vi "viserverUserAccess_getUserNamesSymbols.vi"(0 "ACL in":refnum<k20>, 5 "principal array in":T1[](array[typedef]) {"principal"."ID"."b7" format="%02x"; "principal"."ID"."b6" format="%02x"; "principal"."ID"."b5" format="%02x"; "principal"."ID"."b4" format="%02x"; "principal"."ID"."b3" format="%02x"; "principal"."ID"."b2" format="%02x"; "principal"."ID"."b1" format="%02x"; "principal"."ID"."b0" format="%02x"; "principal"."ID"."b15" format="%02x"; "principal"."ID"."b14" format="%02x"; "principal"."ID"."b13" format="%02x"; "principal"."ID"."b12" format="%02x"; "principal"."ID"."b11" format="%02x"; "principal"."ID"."b10" format="%02x"; "principal"."ID"."b9" format="%02x"; "principal"."ID"."b8" format="%02x"; "domain"."ID"."b7" format="%02x"; "domain"."ID"."b6" format="%02x"; "domain"."ID"."b5" format="%02x"; "domain"."ID"."b4" format="%02x"; "domain"."ID"."b3" format="%02x"; "domain"."ID"."b2" format="%02x"; "domain"."ID"."b1" format="%02x"; "domain"."ID"."b0" format="%02x"; "domain"."ID"."b15" format="%02x"; "domain"."ID"."b14" format="%02x"; "domain"."ID"."b13" format="%02x"; "domain"."ID"."b12" format="%02x"; "domain"."ID"."b11" format="%02x"; "domain"."ID"."b10" format="%02x"; "domain"."ID"."b9" format="%02x"; "domain"."ID"."b8" format="%02x"}, 11 "error in (no error)":errorcluster) -> (4 "ACL out":refnum<k20>, 6 "principal array out":T1[](array[typedef]) {"principal"."ID"."b7" format="%02x"; "principal"."ID"."b6" format="%02x"; "principal"."ID"."b5" format="%02x"; "principal"."ID"."b4" format="%02x"; "principal"."ID"."b3" format="%02x"; "principal"."ID"."b2" format="%02x"; "principal"."ID"."b1" format="%02x"; "principal"."ID"."b0" format="%02x"; "principal"."ID"."b15" format="%02x"; "principal"."ID"."b14" format="%02x"; "principal"."ID"."b13" format="%02x"; "principal"."ID"."b12" format="%02x"; "principal"."ID"."b11" format="%02x"; "principal"."ID"."b10" format="%02x"; "principal"."ID"."b9" format="%02x"; "principal"."ID"."b8" format="%02x"; "domain"."ID"."b7" format="%02x"; "domain"."ID"."b6" format="%02x"; "domain"."ID"."b5" format="%02x"; "domain"."ID"."b4" format="%02x"; "domain"."ID"."b3" format="%02x"; "domain"."ID"."b2" format="%02x"; "domain"."ID"."b1" format="%02x"; "domain"."ID"."b0" format="%02x"; "domain"."ID"."b15" format="%02x"; "domain"."ID"."b14" format="%02x"; "domain"."ID"."b13" format="%02x"; "domain"."ID"."b12" format="%02x"; "domain"."ID"."b11" format="%02x"; "domain"."ID"."b10" format="%02x"; "domain"."ID"."b9" format="%02x"; "domain"."ID"."b8" format="%02x"}, 8 "User/group names":string[](array[string]), 10 "User/group access symbols":i32[](array[numeric]), 15 "error out":errorcluster)   [LabVIEW 2020]
uses:
  <vilib>/Platform/security/user/NI_Security Qualified Domain-Principal Pair.ctl
  <vilib>/Platform/security/user/NI_Security Domain.ctl
  <vilib>/Platform/security/user/NI_Security Identifier.ctl
  <vilib>/Platform/security/user/NI_Security Principal.ctl
  <vilib>/Platform/security/user/NI_Security PrincipalType.ctl
  <vilib>/Platform/SharedPrefPage_SubVIs/viServerUserAccess_user_group_enum.ctl
  <vilib>/Platform/security/user/NI_Security AccessRights_CloseRef.vi
  <vilib>/Platform/security/user/NI_Security ACE_CloseRef.vi
  <resource>/objmgr/Security.rc
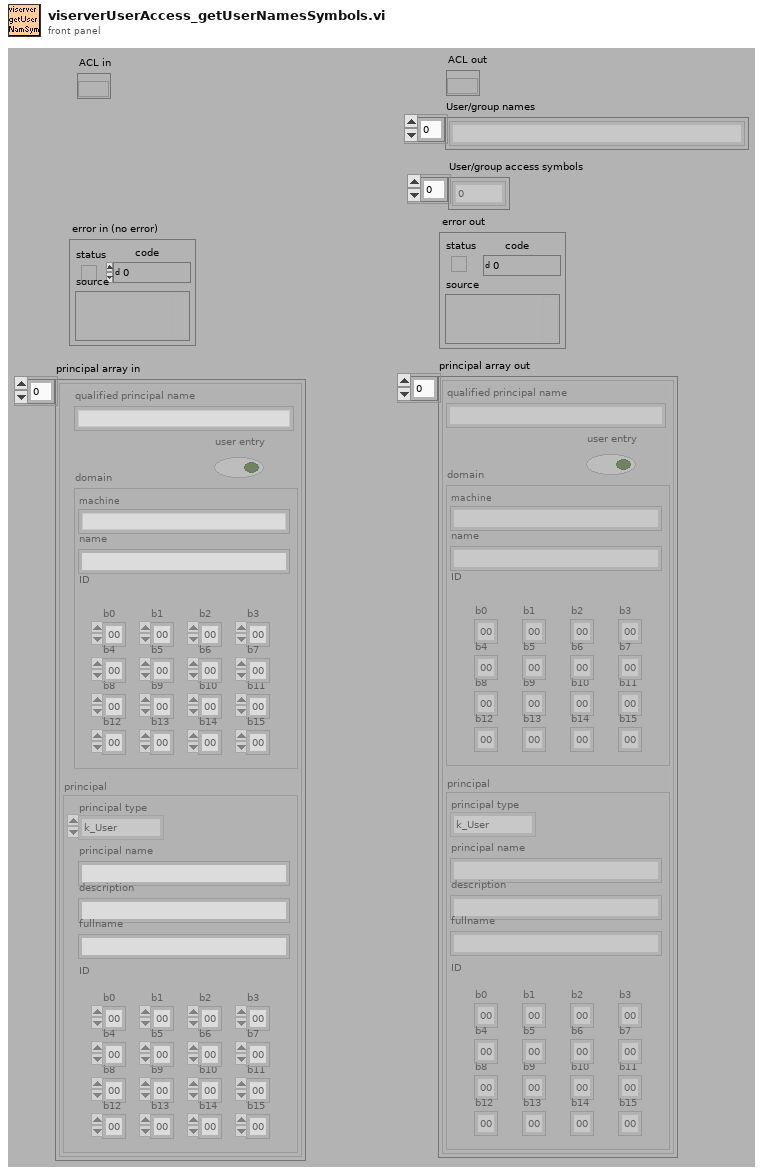
[diagram p1: front panel]
types:
  T1 = typedef "NI_Security Qualified Domain-Principal Pair.ctl" = cluster{"qualified principal name":string, "domain":T2, "principal":T4, "user entry":bool}
  T2 = typedef "NI_Security Domain.ctl" = cluster{"machine":string, "name":string, "ID":T3}
  T3 = typedef "NI_Security Identifier.ctl" = cluster{"b0":u8, "b1":u8, "b2":u8, "b3":u8, "b4":u8, "b5":u8, "b6":u8, "b7":u8, "b8":u8, "b9 ":u8, "b10":u8, "b11":u8, "b12":u8, "b13":u8, "b14":u8, "b15":u8}
  T4 = typedef "NI_Security Principal.ctl" = cluster{"principal type":T5, "principal name":string, "description":string, "fullname":string, "ID":T3}
  T5 = typedef "NI_Security PrincipalType.ctl" = enum16{"k_User", "k_Group"}
  T6 = typedef "viServerUserAccess_user_group_enum.ctl" = enum16{"None", "User - allow", "User - deny", "Group - allow", "Group - deny"}
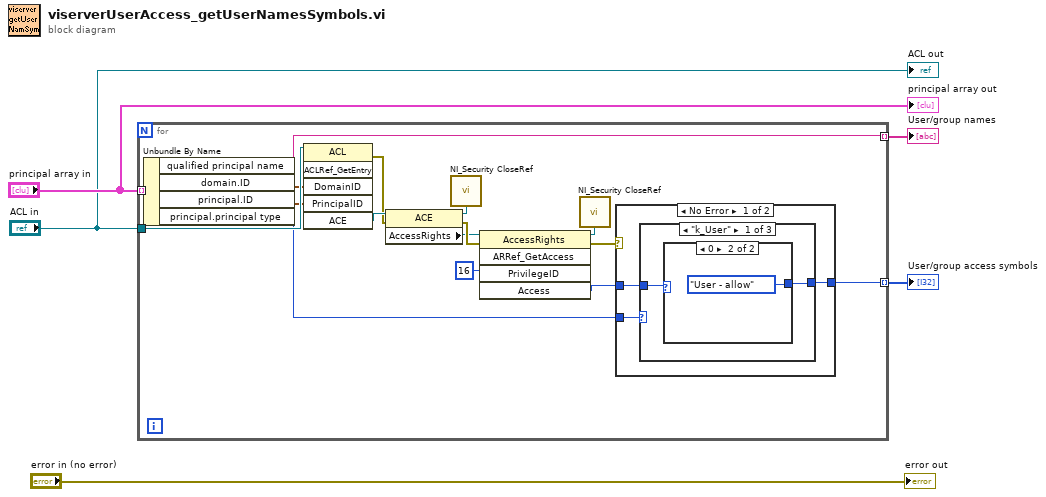
[diagram p0: block diagram]
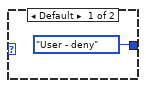
[diagram p2: hidden frame]
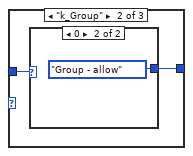
[diagram p3: hidden frame]
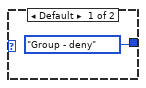
[diagram p4: hidden frame]
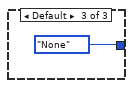
[diagram p5: hidden frame]
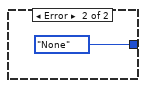
[diagram p6: hidden frame]
diagram:
  n1 = for {
    tunnel: "principal array in" -> [w21] mode=indexing
    tunnel: "ACL in" -> [w20]
    tunnel: [w15] -> w2 mode=indexing
    tunnel: [w7] -> w1 mode=indexing
    n2 = Unbundle By Name(w21) -> ("qualified principal name"=w7:string, "domain.ID"=w9:T3, "principal.ID"=w8:T3, "principal.principal type"=w6:T5)
    n3 = invoke class="ACL" method="ACLRef_GetEntry"(reference=w20, "DomainID"=w9, "PrincipalID"=w8) -> (error out=w12:errorcluster, "ACE"=w14:refnum<k20>)  [unwired: 3 in, 4 out]
    n4 = property class="ACE"(reference=w14, error in=w12) -> (reference out=w13:refnum<k20>, error out=w11:errorcluster, "AccessRights"=w10:refnum<k20>)
    n5 = call-poly <vilib>:"NI_Security CloseRef.vi"("security refnum"=w13) -> ()  [unwired: 10 in, 1 out]
    n6 = invoke class="AccessRights" method="ARRef_GetAccess"(reference=w10, error in=w11, "PrivilegeID"=u32 16) -> (reference out=w18:refnum<k20>, error out=w17:errorcluster, "Access"=w16:u32)  [unwired: 2 in, 2 out]
    n7 = call-poly <vilib>:"NI_Security CloseRef.vi"("security refnum"=w18) -> ()  [unwired: 10 in, 1 out]
    n8 = case shown="No Error" w17 {
      tunnel: w16 -> [w22 _]
      tunnel: [w23 viServerUserAccess_user_group_enum."None" ("User/group allow/deny enum")] -> w15
      tunnel: w6 -> [w24 _]
      frame No Error {
        n9 = case shown="\"k_User\"" w24 {
          tunnel: [w25 w29 viServerUserAccess_user_group_enum."None" ("User/group allow/deny enum")] -> w23
          tunnel: w22 -> [w26 w30 _]
          frame "k_User" {
            n10 = case shown="0" w26 {
              tunnel: [viServerUserAccess_user_group_enum."User - deny" ("User/group allow/deny enum") viServerUserAccess_user_group_enum."User - allow" ("User/group allow/deny enum")] -> w25
              frame Default {
              }
              frame 0 {
              }
            }
          }
          frame "k_Group" {
            n11 = case shown="0" w30 {
              tunnel: [viServerUserAccess_user_group_enum."Group - deny" ("User/group allow/deny enum") viServerUserAccess_user_group_enum."Group - allow" ("User/group allow/deny enum")] -> w29
              frame Default {
              }
              frame 0 {
              }
            }
          }
          frame Default {
          }
        }
      }
      frame Error {
      }
    }
  }
  "User/group names" <- w1
  "User/group access symbols" <- w2
  "error out" <- "error in (no error)"
  "principal array out" <- "principal array in"
  "ACL out" <- "ACL in"
